vi "Ref Top Level.vi"(5 "Offset":refnum<class "Offset.lvclass"> caption="Offset (None)", 6 "Size":refnum<class "Size.lvclass"> caption="Size (Unchanged)", 7 "Alignment":T1={"Horizontal"=enum."Center", "Vertical"=enum."Center"} caption="Alignment (Center, Center)", 8 "Error In":errorcluster) -> (0 "Error Out":errorcluster, 3 "Ref Top Level out":refnum<class "Ref Top Level.lvclass">)   [LabVIEW 2017, in "MGI-Panel Manager.lvlib" / "Ref Top Level.lvclass"]
doc: "Constructs a window positioner that will uses the top level panel's screen position as an anchor.\n\nThe top level panel is automatically determined by the framework.\n\n<B>Alignment:</B> Set the type of alignment\n<B>Offset:</B> Input Offset object.\n<B>Size:</B> Input Size object.\n<B>Error In:</B> Describes error conditions that occur before this node runs.\n\n<B>Top Level Ref Out:</B> A Top Level Reference Position object.\n<B>Error Out:</B> Contains error information.\n\n----\nPlease see the following web address for additional documentation and tutorial information:\nhttp://www.mooregoodideas.com/mgi-panel-manager/\n\nAuthor: Derek Trepanier\n\nCopyright (c) 2018, Moore Good Ideas, Inc.\n\nAll rights reserved.\n\nRedistribution and use in source and binary forms, with or without modification, are permitted provided that the following conditions are met:\n\n * Redistributions of source code must retain the above copyright notice, this list of conditions and the following disclaimer.\n * Redistributions in binary form must reproduce the above copyright notice, this list of conditions and the following disclaimer in the documentation and/or other materials provided with the distribution.\n * Neither the name of Moore Good Ideas, Inc. nor the names of its contributors may be used to endorse or promote products derived from this software without specific prior written permission.\n\nTHIS SOFTWARE IS PROVIDED BY THE COPYRIGHT HOLDERS AND CONTRIBUTORS \"AS IS\" AND ANY EXPRESS OR IMPLIED WARRANTIES, INCLUDING, BUT NOT LIMITED TO, THE IMPLIED WARRANTIES OF MERCHANTABILITY AND FITNESS FOR A PARTICULAR PURPOSE ARE DISCLAIMED. IN NO EVENT SHALL THE COPYRIGHT OWNER OR CONTRIBUTORS BE LIABLE FOR ANY DIRECT, INDIRECT, INCIDENTAL, SPECIAL, EXEMPLARY, OR CONSEQUENTIAL DAMAGES (INCLUDING, BUT NOT LIMITED TO, PROCUREMENT OF SUBSTITUTE GOODS OR SERVICES; LOSS OF USE, DATA, OR PROFITS; OR BUSINESS INTERRUPTION) HOWEVER CAUSED AND ON ANY THEORY OF LIABILITY, WHETHER IN CONTRACT, STRICT LIABILITY, OR TORT (INCLUDING NEGLIGENCE OR OTHERWISE) ARISING IN ANY WAY OUT OF THE USE OF THIS SOFTWARE, EVEN IF ADVISED OF THE POSSIBILITY OF SUCH DAMAGE."
uses:
  Ref Top Level.lvclass
  Reference Position.lvclass
  Vertical Alignment.ctl
  Horizontal Alignment.ctl
  Alignment.ctl
  Offset/Offset.lvclass
  Size/Size.lvclass
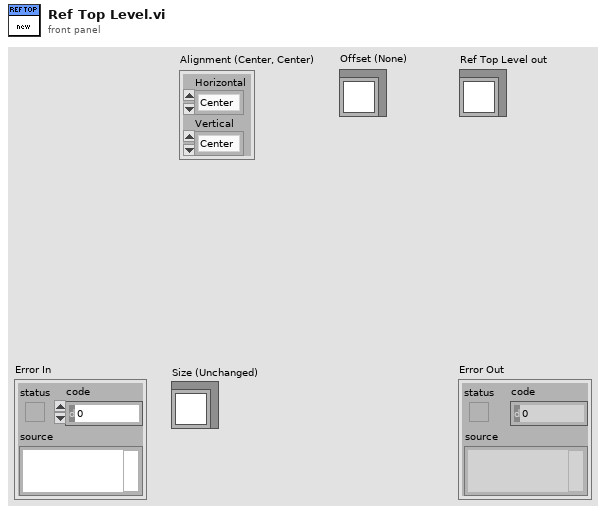
[diagram p1: front panel]
types:
  T1 = typedef "MGI-Panel Manager.lvlib/Reference Position.lvclass/Alignment.ctl" = cluster{"Horizontal":T2, "Vertical":T3}
  T2 = typedef "MGI-Panel Manager.lvlib/Reference Position.lvclass/Horizontal Alignment.ctl" = enum16{"Left", "Center", "Right"}
  T3 = typedef "MGI-Panel Manager.lvlib/Reference Position.lvclass/Vertical Alignment.ctl" = enum16{"Top", "Center", "Bottom"}
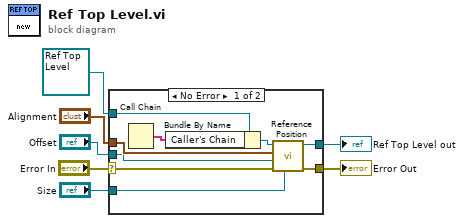
[diagram p0: block diagram]
diagram:
  n1 = case shown="No Error" "Error In" {
    selector: "Error In" -> [w11 w18]
    tunnel: [w10 w18] -> w6
    tunnel: [w14 w17] -> w4
    tunnel: refnum<class "Ref Top Level.lvclass"> refnum ("Ref Top Level in") -> [w16 w17]
    tunnel: "Alignment" -> [w13 _]
    tunnel: "Offset" -> [w12 _]
    tunnel: "Size" -> [w8 _]
    frame No Error {
      n2 = Call Chain() -> (call chain=w9:string[])
      n3 = Bundle By Name(cluster=w16, "Caller's Chain"=w9) -> (w15:refnum<class "Ref Top Level.lvclass">)
      n4 = call "Reference Position.vi"("Size"=w8, "error in (no error)"=w11, "Offset"=w12, "Alignment"=w13, "Reference Position in"=w15) -> ("error out"=w10:errorcluster, "Reference Position out"=w14:refnum<class "Ref Top Level.lvclass">)  [unwired: 5 in]
    }
    frame Error {
    }
  }
  "Error Out" <- w6
  "Ref Top Level out" <- w4
